vi "Read Start Index.vi"(8 "error in (no error)":errorcluster, 11 "Set Lengths Msg in":refnum<class "Set Lengths Msg.lvclass">) -> (0 "error out":errorcluster, 2 "Start Index":i32, 3 "Set Lengths Msg out":refnum<class "Set Lengths Msg.lvclass">)   [LabVIEW 2017, in "BNT_DAQmx.lvlib" / "Set Lengths Msg.lvclass"]
uses:
  Set Lengths Msg.lvclass
  Set Lengths Msg.lvclass/Set Lengths Msg.ctl
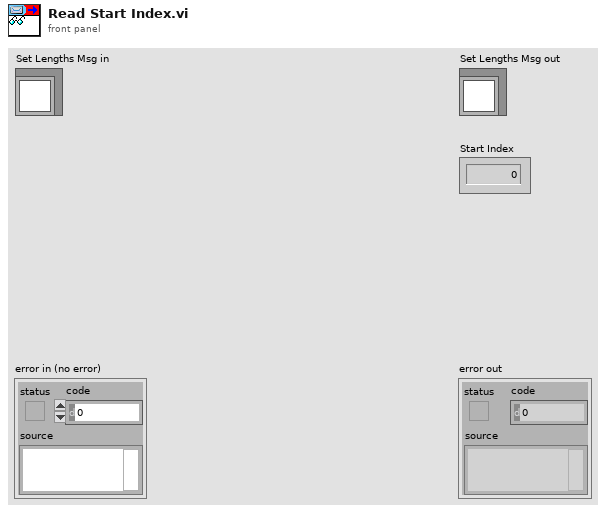
[diagram p1: front panel]
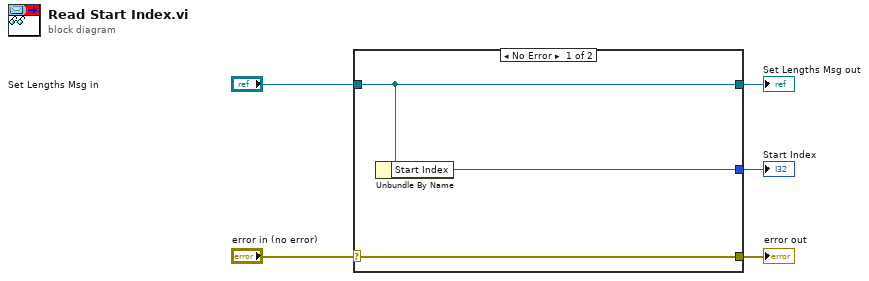
[diagram p0: block diagram]
diagram:
  n1 = case shown="No Error" "error in (no error)" {
    selector: "error in (no error)" -> [w8 w9]
    tunnel: [w8 w9] -> w4
    tunnel: [w7 w10] -> w2
    tunnel: "Set Lengths Msg in" -> [w7 w10]
    tunnel: [w6 _] -> w1
    frame No Error {
      n2 = Unbundle By Name(w7) -> ("Start Index"=w6:i32)
    }
    frame Error {
    }
  }
  "error out" <- w4
  "Set Lengths Msg out" <- w2
  "Start Index" <- w1
